vi "front pannel origin.vi"(8 "error in":errorcluster) -> (0 "error out":errorcluster)   [LabVIEW 2020]
uses:
  <vilib>/Utility/miscctls.llb/LVPointTypeDef.ctl
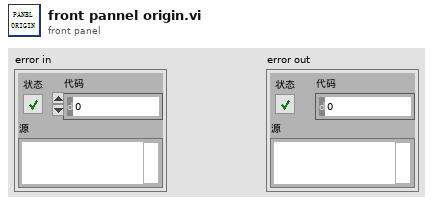
[diagram p1: front panel]
types:
  T1 = typedef "LVPointTypeDef.ctl" = cluster{"Horizontal":i16, "Vertical":i16}
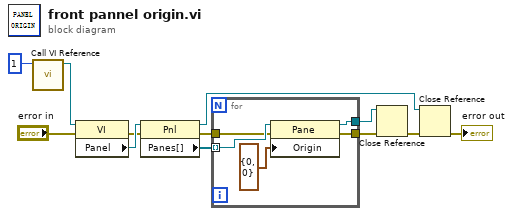
[diagram p0: block diagram]
diagram:
  n1 = call "Call VI Reference.vi"("last level"=1 ("上层调用索引")) -> ("vi reference out"=w11:refnum<vi>)  [unwired: 9 in, 1 out]
  n2 = property class="VI"(reference=w11, error in="error in") -> (error out=w7:errorcluster, "Panel"=w10:refnum<vi>)  [unwired: 1 out]
  n3 = property class="Pnl"(reference=w10, error in=w7) -> (reference out=w3:refnum<vi>, error out=w6:errorcluster, "Panes[]"=w9:refnum<vi>[])
  n4 = for {
    tunnel: w9 -> [w17] mode=indexing
    tunnel: [w14] -> w4
    tunnel: w6 -> [w16]
    tunnel: [w15] -> w5
    n5 = property class="Pane"(reference=w17, error in=w16, "Origin"=T1 {"Horizontal"=0, "Vertical"=0} ("原点")) -> (reference out=w14:refnum<vi>, error out=w15:errorcluster)
  }
  n6 = Close Reference(reference=w4, error in (no error)=w5) -> (error out=w2:errorcluster)
  n7 = Close Reference(reference=w3, error in (no error)=w2) -> (error out=→"error out":errorcluster)
